vi "Map_-180_179.vi"(1 "Angle In":i32) -> (0 "-180 <= Angle out <180":i32)   [LabVIEW 2011]
doc: "Takes an integer angle and maps it to a value between -180 and 179, inclusive."
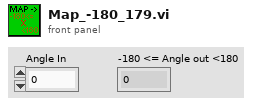
[diagram p1: front panel]
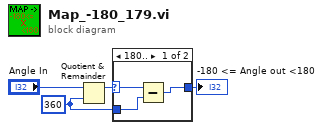
[diagram p0: block diagram]
diagram:
  w4 = 360 ("y")
  n1 = Quotient & Remainder(x="Angle In", y=w4) -> (x-y*floor(x/y)=w2:i32)  [unwired: 1 out]
  n2 = case shown="180.." w2 {
    selector: w2 -> [w7 w8]
    tunnel: [w5 w8] -> w3
    tunnel: w4 -> [w6 _]
    frame 180.. {
      n3 = Subtract(x=w7, y=w6) -> (x-y=w5:i32)
    }
    frame ..179 {
    }
  }
  "-180 <= Angle out <180" <- w3
